vi "LoadGlobais2.vi"(8 "error in (no error)":errorcluster, 10 "Mecanismo":string, 11 "Device in":refnum<class "Device.lvclass">) -> (0 "error out":errorcluster, 2 "Resp":string, 3 "Device out":refnum<class "Device.lvclass">)   [LabVIEW 2018, in "Device.lvclass"]
uses:
  Device.lvclass
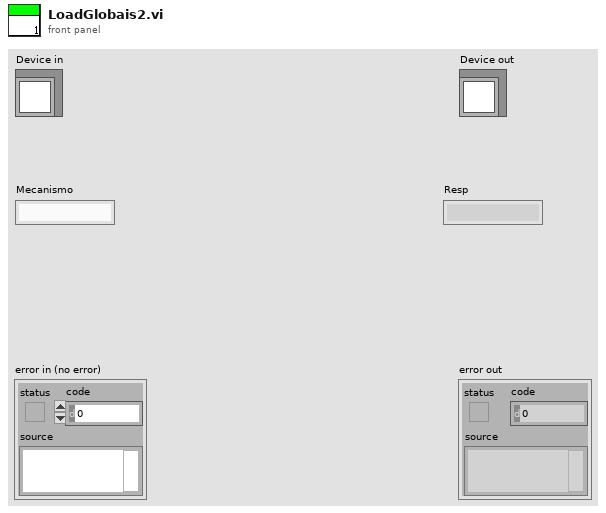
[diagram p1: front panel]
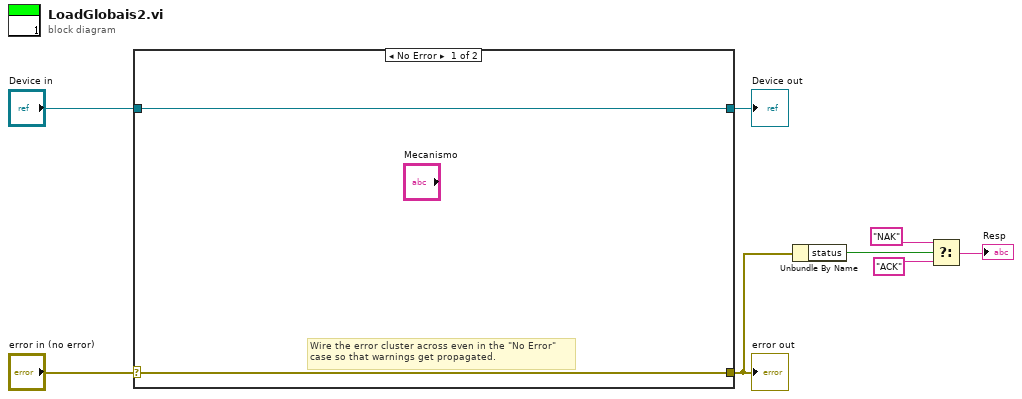
[diagram p0: block diagram]
diagram:
  n1 = case shown="No Error" "error in (no error)" {
    selector: "error in (no error)" -> [w9 w12]
    tunnel: [w9 w12] -> w1
    tunnel: [w10 w11] -> w6
    tunnel: "Device in" -> [w10 w11]
    frame No Error {
      # "Wire the error cluster across even in the \"No Error\"\ncase so that warnings get propagated."
    }
    frame Error {
    }
  }
  "error out" <- w1
  "Device out" <- w6
  n2 = Unbundle By Name(w1) -> ("status"=w5:bool)
  n3 = Select(t="NAK", s=w5, f="ACK") -> (s? t:f=→"Resp":string)
